vi "get_space_usage.vi"(8 "error in (no error)":errorcluster) -> (0 "error out":errorcluster, 1 "remaining":dbl, 2 "allocated":dbl, 3 "used":dbl)   [LabVIEW 2015, in "lv-dropbox.lvlib" / "v2.lvlib"]
uses:
  v2.lvlib
  <vilib>/httpClient/POSTBuffer.vi
  <vilib>/httpClient/LabVIEWHTTPClient.lvlib
  lv-dropbox.lvlib
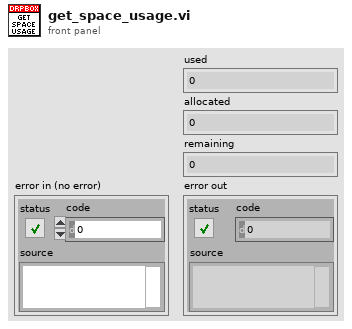
[diagram p1: front panel]
types:
  T1 = cluster{"used":dbl, "allocation":cluster{".tag":string, "allocated":dbl}}
  T2 = typedef "LabVIEWHTTPClient.lvlib/ClientHandle.ctl" = refnum<k1>
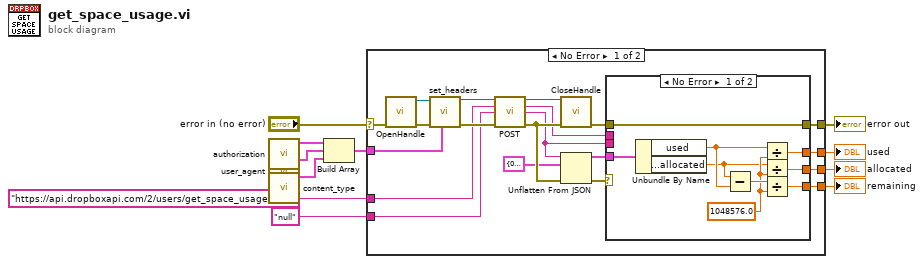
[diagram p0: block diagram]
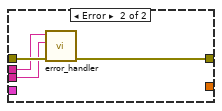
[diagram p2: hidden frame]
diagram:
  n1 = call "authorization.vi"() -> ("header"=w6:cluster{"header":string, "value":string})  [unwired: 11 in]
  n2 = call "user_agent.vi"() -> ("header"=w5:cluster{"header":string, "value":string})  [unwired: 11 in]
  n3 = call "content_type.vi"() -> ("header"=w7:cluster{"header":string, "value":string})  [unwired: 11 in]
  n4 = Build Array(w6, w5, w7) -> (w8:cluster{"header":string, "value":string}[])
  n5 = case shown="No Error" "error in (no error)" {
    selector: "error in (no error)" -> [w24 w45]
    tunnel: "https://api.dropboxapi.com/2/users/get_space_usage" ("url") -> [w29 _]
    tunnel: "null" ("buffer") -> [w28 _]
    tunnel: w8 -> [w22 _]
    tunnel: [w14 w45] -> w4
    tunnel: [w19 _] -> w3
    tunnel: [w18 _] -> w2
    tunnel: [w17 _] -> w1
    frame No Error {
      n6 = call <vilib>:"OpenHandle.vi"("error in (no error)"=w24) -> ("client handle out"=w25:T2, "error out"=w23:errorcluster)  [unwired: 13 in]
      n7 = call "set_headers.vi"("header_value []"=w22, "error in (no error)"=w23, "client_handle in"=w25) -> ("error out"=w30:errorcluster, "client_handle out"=w21:T2)  [unwired: 7 in]
      n8 = call-poly <vilib>:"POST.vi"("client handle"=w21, "url"=w29, "buffer"=w28, "error in (no error)"=w30) -> ("client handle out"=w20:T2, "headers"=w13:string, "body"=w12:string, "error out"=w31:errorcluster)  [unwired: 8 in]
      n9 = call <vilib>:"CloseHandle.vi"("client handle"=w20, "error in (no error)"=w31) -> ("error out"=w15:errorcluster)  [unwired: 13 in]
      n10 = Unflatten From JSON(JSON string=w12, type and defaults=T1 {"used"=0.0, "allocation"={".tag"="", "allocated"=0.0}} ("value"), error in (no error)=w31) -> (value=w26:T1, error out=w16:errorcluster)  [unwired: 4 in]
      n11 = case shown="No Error" w16 {
        tunnel: w26 -> [w38 _]
        tunnel: [w35 _] -> w19
        tunnel: [w34 _] -> w18
        tunnel: [w33 _] -> w17
        tunnel: w15 -> [w32 w44]
        tunnel: [w32 w41] -> w14
        tunnel: w13 -> [_ w43]
        tunnel: w12 -> [_ w42]
        frame No Error {
          w39 = 1048576.0 ("x")
          n12 = Unbundle By Name(w38) -> ("used"=w37:dbl, "allocation.allocated"=w36:dbl)
          n13 = Subtract(x=w36, y=w37) -> (x-y=w40:dbl)
          n14 = Divide(x=w37, y=w39) -> (x/y=w35:dbl)
          n15 = Divide(x=w36, y=w39) -> (x/y=w34:dbl)
          n16 = Divide(x=w40, y=w39) -> (x/y=w33:dbl)
        }
        frame Error {
          n17 = call "error_handler.vi"("error in (no error)"=w44, "body"=w42, "headers"=w43) -> ("error out"=w41:errorcluster)  [unwired: 8 in]
        }
      }
    }
    frame Error {
    }
  }
  "error out" <- w4
  "used" <- w3
  "remaining" <- w1
  "allocated" <- w2
